vi "DLTS - setup DAQ (SubVI).vi"(4 "No. samples":i32=1000000, 5 "post trigger delay":dbl format="%#_13g", 6 "No. repetitions (avg)":i32=2, 7 "Selected device":string, 8 "error in (no error)":errorcluster, 9 "AUX offset":dbl, 10 "AUX scale":dbl, 11 "Handle in":T1 {"Handle" format="0x%08x"; "Conn" format="0x%08x"}) -> (0 "error out":errorcluster, 2 "ModHandle Out":T2 {"ModHandle" format="0x%08x"; "Conn" format="0x%08x"}, 3 "Handle Out":T1 {"Handle" format="0x%08x"; "Conn" format="0x%08x"})   [LabVIEW 2019]
doc: "Configures DLTS data acquisition"
uses:
  <instrlib>/Zurich Instruments LabOne/Public/Modules/ziTypeModHandle.ctl
  <instrlib>/Zurich Instruments LabOne/Public/ziTypeHandle.ctl
  <instrlib>/Zurich Instruments LabOne/Public/Modules/ziTypeModEnum.ctl
  <instrlib>/Zurich Instruments LabOne/Public/Modules/ziModSetValueBinaryArray.vi
  <instrlib>/Zurich Instruments LabOne/Public/Modules/ziModSetValueDoubleArray.vi
  <instrlib>/Zurich Instruments LabOne/Zurich Instruments LabOne.lvlib
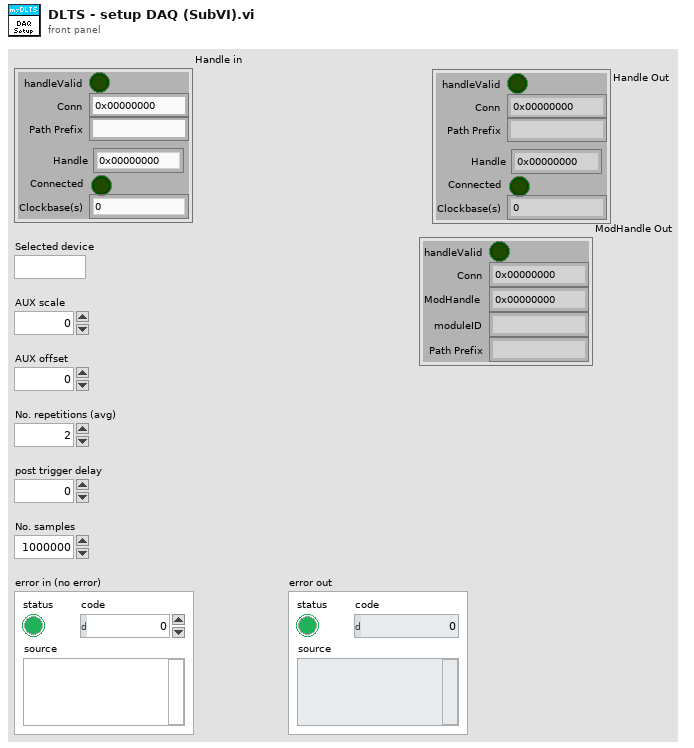
[diagram p1: front panel]
types:
  T1 = typedef "Zurich Instruments LabOne.lvlib/ziTypeHandle.ctl" = cluster{"handleValid":bool, "Conn":u64, "Path Prefix":string, "Handle":u64, "Connected":bool, "Clockbase(s)":dbl}
  T2 = typedef "Zurich Instruments LabOne.lvlib/ziTypeModHandle.ctl" = cluster{"handleValid":bool, "Conn":u64, "ModHandle":u64, "moduleID":string, "Path Prefix":string}
  T3 = typedef "Zurich Instruments LabOne.lvlib/ziTypeModEnum.ctl" = u16
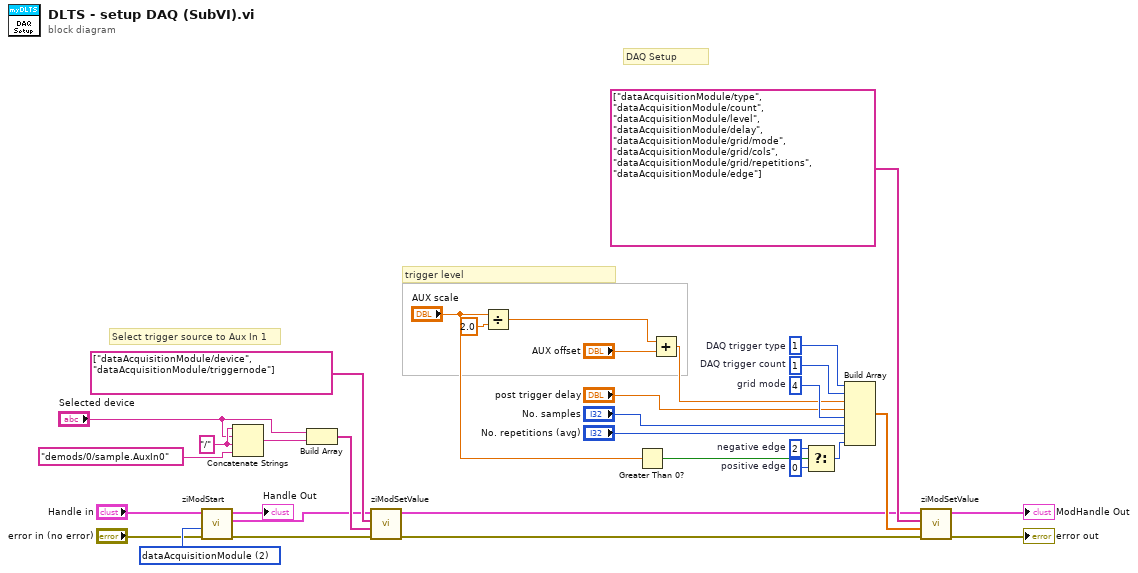
[diagram p0: block diagram]
diagram:
  w29 = 4  # grid mode
  w28 = 1  # DAQ trigger count
  w27 = 1  # DAQ trigger type
  w21 = "/" ("string")
  w15 = T3 2 items=["sweep", "scopeModule", "dataAcquisitionModule", "pidAdvisor", "awgModule", "impedanceModule", "multiDeviceSyncModule", "zoomFFT", "trigger", "deviceSettings", "record", "precompensationAdvisor"] ("module Id")
  w9 = 0  # positive edge
  w8 = 2  # negative edge
  # "Select trigger source to Aux In 1"
  # "DAQ Setup"
  # "trigger level"
  n1 = call <instrlib>:"ziModStart.vi"("Error In"="error in (no error)", "module Id"=w15, "Handle In"="Handle in") -> ("Error Out"=w17:errorcluster, "ModHandle Out"=w16:T2, "Handle Out"=→"Handle Out":T1)  [unwired: 6 in]
  n2 = Concatenate Strings(w21, "Selected device", w21, "demods/0/sample.AuxIn0" ("string")) -> (w20:string)
  n3 = Build Array("Selected device", w20) -> (w19:string[])
  n4 = call-poly <instrlib>:"ziModSetValue.vi"("Error In"=w17, "Values"=w19, "Paths"=string[] ["dataAcquisitionModule/device", "dataAcquisitionModule/triggernode"], "ModHandle In"=w16) -> ("Error Out"=w24:errorcluster, "ModHandle Out"=w23:T2)  [unwired: 6 in]
  n5 = Divide(x="AUX scale", y=2.0) -> (x/y=w3:dbl)
  n6 = Greater Than 0?(x="AUX scale") -> (x > 0?=w7:bool)
  n7 = Add(x=w3, y="AUX offset") -> (x+y=w4:dbl)
  n8 = Select(t=w8, s=w7, f=w9) -> (s? t:f=w10:i32)
  n9 = Build Array(w27, w28, w4, "post trigger delay", w29, "No. samples", "No. repetitions (avg)", w10) -> (w26:dbl[])
  n10 = call-poly <instrlib>:"ziModSetValue.vi"("Error In"=w24, "Values"=w26, "Paths"=string[] ["dataAcquisitionModule/type", "dataAcquisitionModule/count", "dataAcquisitionModule/level", "dataAcquisitionModule/delay", "dataAcquisitionModule/grid/mode", "dataAcquisitionModule/grid/cols", "dataAcquisitionModule/grid/repetitions", "dataAcquisitionModule/edge"], "ModHandle In"=w23) -> ("Error Out"=→"error out":errorcluster, "ModHandle Out"=→"ModHandle Out":T2)  [unwired: 6 in]
